vi "MutationHistoryGUI.vi"(10 "Title":string, 11 "LVClass path":path) -> ()   [LabVIEW 2019, in "MutationHistoryGUI.lvlib"]
uses:
  MutationHistoryGUI.lvlib
  <userlib>/Blue Origin/BlueVariantView/API/Typedefs/Options.ctl
  <resource>/Framework/Providers/BlueSerializationProviderShared/UserCommentToVersion.vi
  <userlib>/Blue Origin/BlueVariantView/BlueVariantView.lvlib
panel:
  in  "Listbox":i32(listbox)
  out "Tree":string(tree)
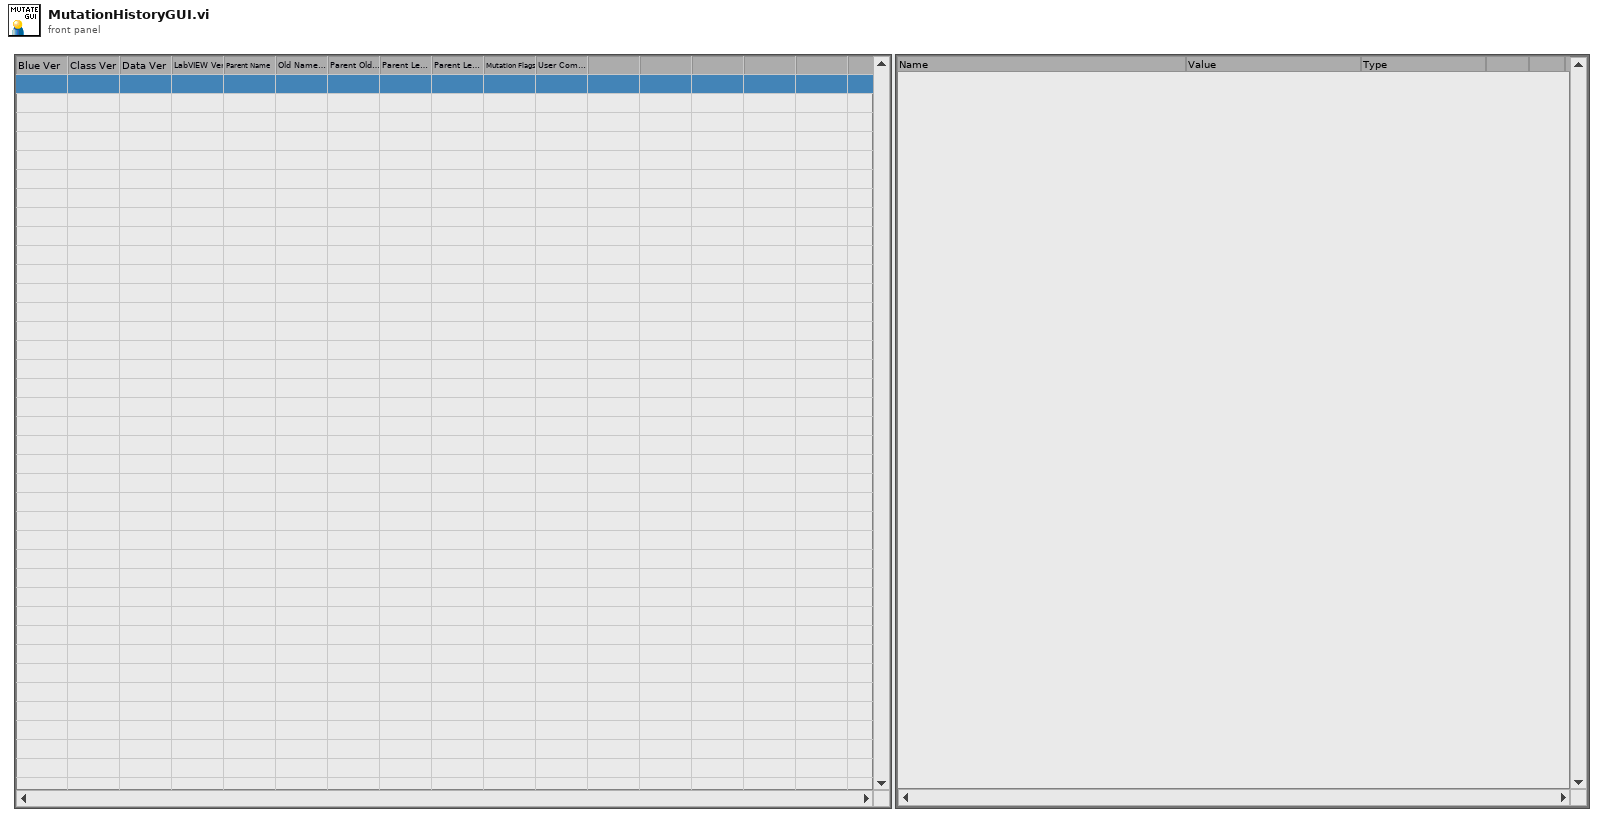
[diagram p1: front panel]
types:
  T1 = typedef "Edit LVLibs.lvlib/Mutation History.ctl" = T2[]
  T2 = typedef "Edit LVLibs.lvlib/Mutation Record.ctl" = cluster{"Library Version":T3, "Old Name Index":u8, "Class Default Data":variant, "Cluster Order Map":u32[], "Parent Name":string, "Parent Path":path, "LabVIEW Version":u32, "User Comments":string, "Mutation Flags":u8, "Parent Old Name Index":u8, "Parent Levels Added":u16, "Parent Levels Removed":u16}
  T3 = typedef "Edit LVLibs.lvlib/LibVersion.ctl" = cluster{"Major":u16, "Minor":u16, "Fix":u16, "Build":u16}
  T4 = enum16{"No Scaling", "Scale All Objects", "Scale Single Object"}
  T5 = typedef "BlueVariantView.lvlib/Options.ctl" = cluster{"Colorize?":bool}
  T6 = typedef "LVPoint32TypeDef.ctl" = cluster{"Horizontal":i32, "Vertical":i32}
  T7 = typedef "LVRowAndColumnTypeDef.ctl" = cluster{"Row":i32, "Column":i32}
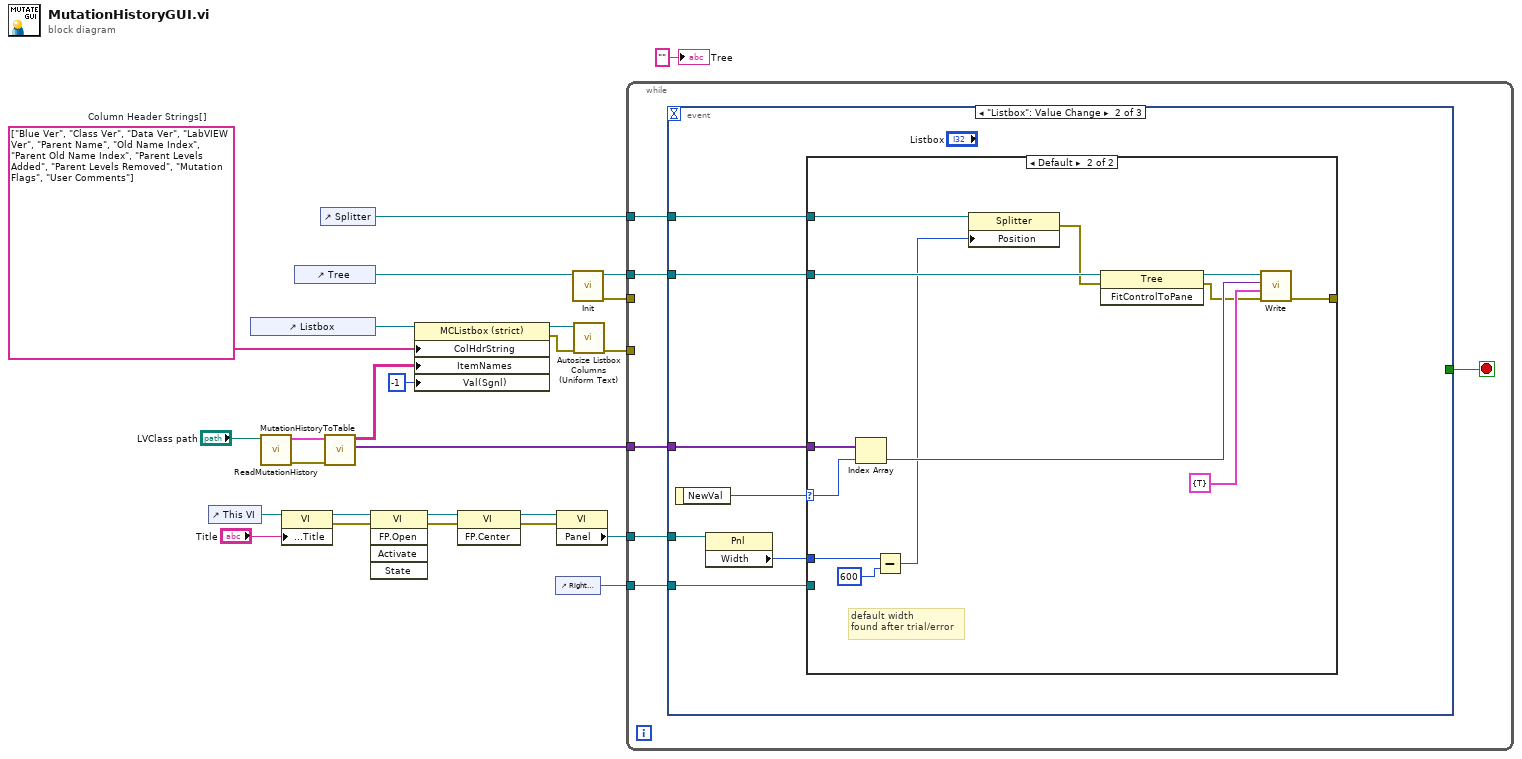
[diagram p0: block diagram]
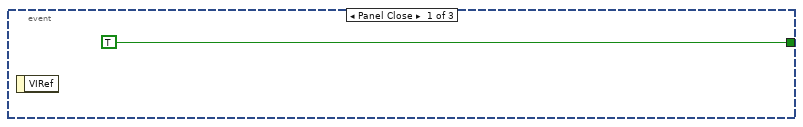
[diagram p2: hidden frame]
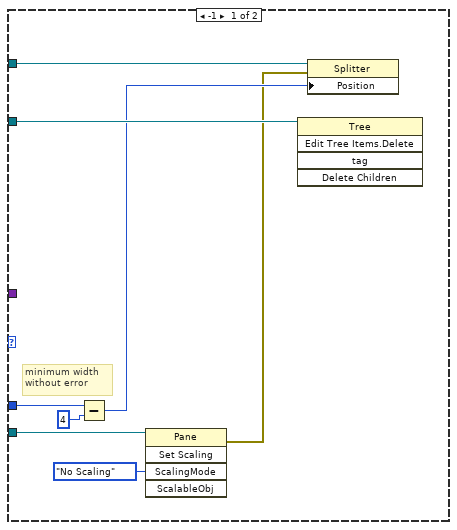
[diagram p3: hidden frame]
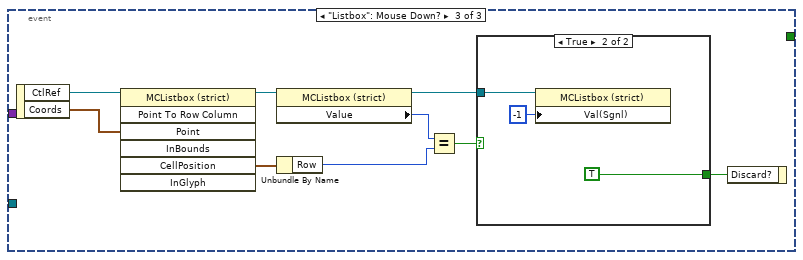
[diagram p4: hidden frame]
diagram:
  w21 = string[] ["Blue Ver", "Class Ver", "Data Ver", "LabVIEW Ver", "Parent Name", "Old Name Index", "Parent Old Name Index", "Parent Levels Added", "Parent Levels Removed", "Mutation Flags", "User Comments"]  # Column Header Strings[]
  n1 = control-ref of="This VI"() -> (w26:refnum<vi>)
  n2 = control-ref of="Listbox"() -> (w24:refnum<vi>)
  n3 = call "ReadMutationHistory.vi"("LVClass path"="LVClass path") -> ("error out"=w1:errorcluster, "Mutation History"=w2:T1)  [unwired: 7 in, 2 out]
  n4 = property class="VI"(reference=w26, "Front Panel.Title"="Title") -> (reference out=w9:refnum<vi>, error out=w6:errorcluster)  [unwired: 1 in]
  n5 = control-ref of="Tree"() -> (w19:refnum<vi>)
  n6 = control-ref of="Splitter"() -> (w12:refnum<vi>)
  n7 = call "MutationHistoryToTable.vi"("error in (no error)"=w1, "Mutation History"=w2) -> ("Class Default Data"=w13:variant[], "Table"=w14:string[][])  [unwired: 8 in]
  n8 = invoke class="VI" method="FP.Open"(reference=w9, error in=w6) -> (reference out=w8:refnum<vi>, error out=w7:errorcluster)  [unwired: 3 in, 3 out]
  n9 = property class="MCListbox (strict)"(reference=w24, "ColHdrString"=w21, "ItemNames"=w14, "Val(Sgnl)"=-1 ("Value (Signaling)")) -> (reference out=w23:refnum<vi>, error out=w22:errorcluster)  [unwired: 1 in]
  n10 = invoke class="VI" method="FP.Center"(reference=w8, error in=w7) -> (reference out=w4:refnum<vi>, error out=w5:errorcluster)  [unwired: 1 in, 1 out]
  n11 = control-ref of="Right Pane"() -> (w11:refnum<vi>)
  n12 = property class="VI"(reference=w4, error in=w5) -> ("Panel"=w10:refnum<vi>)  [unwired: 2 out]
  n13 = call <userlib>:"Init.vi"("Tree in"=w19) -> ("error out"=w17:errorcluster, "Tree out"=w18:refnum<vi>)  [unwired: 9 in]
  n14 = call "Autosize Listbox Columns (Uniform Text).vi"("error in (no error)"=w22, "Table Ref"=w23) -> ("error out"=w20:errorcluster)  [unwired: 4 in, 1 out]
  n15 = while {
    tunnel: w20 -> [_]
    tunnel: w13 -> [w31]
    tunnel: w18 -> [w30]
    tunnel: w17 -> [_]
    tunnel: w12 -> [w29]
    tunnel: w10 -> [w28]
    tunnel: w11 -> [w27]
    stop <- w32 stop-if-true
    n16 = event shown="[1] \"Listbox\": Value Change" {
      selector: _ -> [_ _ _]
      dyn-events: _ -> [_ _ _]
      timeout: _ -> [_ _ _]
      tunnel: [TRUE _ _] -> w32
      tunnel: w31 -> [_ w40 _]
      tunnel: w30 -> [_ w38 _]
      tunnel: w29 -> [_ w34 _]
      tunnel: w28 -> [_ w36 _]
      tunnel: w27 -> [_ w37 _]
      event Panel Close {
        n17 = event-data() -> ()  [unwired: 1 in, 1 out]
      }
      event "Listbox": Value Change {
        n18 = event-data() -> ("NewVal"=w39:i32)  [unwired: 1 in]
        n19 = property class="Pnl"(reference=w36) -> ("Width"=w35:u32)  [unwired: 1 in, 2 out]
        n20 = case shown="Default" w39 {
          selector: w39 -> [_ w60]
          tunnel: w40 -> [_ w61]
          tunnel: w38 -> [w48 w57]
          tunnel: w37 -> [w46 _]
          tunnel: w35 -> [w44 w54]
          tunnel: w34 -> [w43 w53]
          tunnel: [_ w49] -> _
          frame -1 {
            # "minimum width\nwithout error"
            n21 = Subtract(x=w44, y=u32 4 ("Splitter Position")) -> (x-y=w42:u32)
            n22 = invoke class="Pane" method="Set Scaling"(reference=w46, "ScalingMode"=T4."No Scaling" ("Scaling Mode")) -> (error out=w41:errorcluster)  [unwired: 3 in, 4 out]
            n23 = invoke class="Tree" method="Edit Tree Items.Delete"(reference=w48) -> ()  [unwired: 4 in, 5 out]
            n24 = property class="Splitter"(reference=w43, error in=w41, "Position"=w42) -> ()  [unwired: 2 out]
          }
          frame Default {
            # "default width\nfound after trial/error"
            n25 = Index Array(array=w61, index=w60) -> (element=w59:variant)
            n26 = Subtract(x=w54, y=u32 600 ("Splitter Position")) -> (x-y=w52:u32)
            n27 = property class="Splitter"(reference=w53, "Position"=w52) -> (error out=w51:errorcluster)  [unwired: 1 in, 1 out]
            n28 = invoke class="Tree" method="FitControlToPane"(reference=w57, error in=w51) -> (reference out=w56:refnum<vi>, error out=w50:errorcluster)  [unwired: 1 in, 1 out]
            n29 = call <userlib>:"Write.vi"("error in (no error)"=w50, "Options"=T5 {"Colorize?"=TRUE}, "Anything"=w59, "Tree in"=w56) -> ("error out"=w49:errorcluster)  [unwired: 6 in, 1 out]
          }
        }
      }
      event "Listbox": Mouse Down? {
        n30 = event-data() -> ("CtlRef"=w64:refnum<vi>, "Coords"=w63:T6)  [unwired: 1 in]
        n31 = invoke class="MCListbox (strict)" method="Point To Row Column"(reference=w64, "Point"=w63) -> (reference out=w69:refnum<vi>, "CellPosition"=w70:T7)  [unwired: 5 in, 5 out]
        n32 = property class="MCListbox (strict)"(reference=w69) -> (reference out=w65:refnum<vi>, "Value"=w68:i32)  [unwired: 1 in, 1 out]
        n33 = Unbundle By Name(w70) -> ("Row"=w67:i32)
        n34 = Equal?(x=w68, y=w67) -> (x = y?=w66:bool)
        n35 = case shown="True" w66 {
          tunnel: w65 -> [_ w73]
          tunnel: [_ TRUE ("Discard?")] -> w62
          frame False {
          }
          frame True {
            n36 = property class="MCListbox (strict)"(reference=w73, "Val(Sgnl)"=-1 ("Value (Signaling)")) -> ()  [unwired: 1 in, 2 out]
          }
        }
        n37 = event-data("Discard?"=w62) -> ()  [unwired: 1 in, 1 out]
      }
    }
  }
  "Tree" <- "" ("Tree")
